vi "EOL TCP Connection Manager.vi"(8 "error in":errorcluster, 10 "VI Ref":refnum<vi>, 11 "thread queue":refnum<queue>) -> (0 "error out":errorcluster)   [LabVIEW 2012, in "tcp connection.lvclass"]
doc: "acts as a server for a single networked hmi"
uses:
  classes/connection/tcp connection.lvclass
  classes/server side connection/tcp server connection.lvclass
  typedefs/tcp connection info.ctl
  typedefs/connection type.ctl
  interthread comms/typedefs/app type.ctl
  typedefs/interapp tx message request.ctl
  interthread comms/typedefs/interthread message.ctl
  typedefs/interapp message.ctl
  typedefs/interthread get connection status message.ctl
  typedefs/interthread connection status response.ctl
  interthread comms/typedefs/HMI PC thread IDs.ctl
  typedefs/interapp message actions.ctl
  interthread comms/typedefs/state queue fglbl actions.ctl
  interthread comms/typedefs/station cDAQ thread IDs.ctl
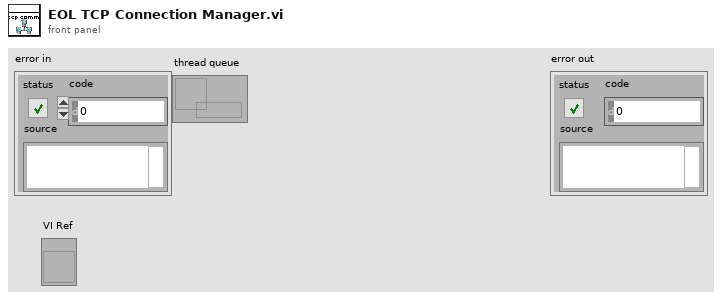
[diagram p1: front panel]
types:
  T1 = typedef "tcp connection info.ctl" = cluster{"server ip address":string, "server port":i32, "connection type":T2}
  T2 = typedef "connection type.ctl" = enum16{"client", "server"}
  T3 = cluster{"connections":refnum<class "tcp connection.lvclass">[]}
  T4 = typedef "station cDAQ thread IDs.ctl" = enum16{"cDAQ main", "analog input", "eol test exe", "nvh test exe", "tcp comms"}
  T5 = typedef "interapp message actions.ctl" = enum16{"init", "request message tx"}
  T6 = typedef "interthread message.ctl" = cluster{"destination state":string, "data":variant}
  T7 = typedef "HMI PC thread IDs.ctl" = enum16{"hmi main", "file output", "tcp comms", "NVH process"}
  T8 = typedef "state queue fglbl actions.ctl" = enum16{"init queues", "get queue ref", "destroy queues"}
  T9 = typedef "interthread get connection status message.ctl" = cluster{"tcp connection info":T1, "reply-to state":string, "reply-to thread":string, "reply-to app":T10}
  T10 = typedef "app type.ctl" = enum16{"PC", "cDAQ", "AuditHMI"}
  T11 = typedef "interthread connection status response.ctl" = cluster{"tcp connection info":T1, "connected":bool}
  T12 = typedef "interapp tx message request.ctl" = cluster{"destination app":T10, "destination thread":string, "tcp connection info":T1, "message":T6}
  T13 = typedef "interapp message.ctl" = cluster{"destination app":T10, "destination thread":string, "message":T6}
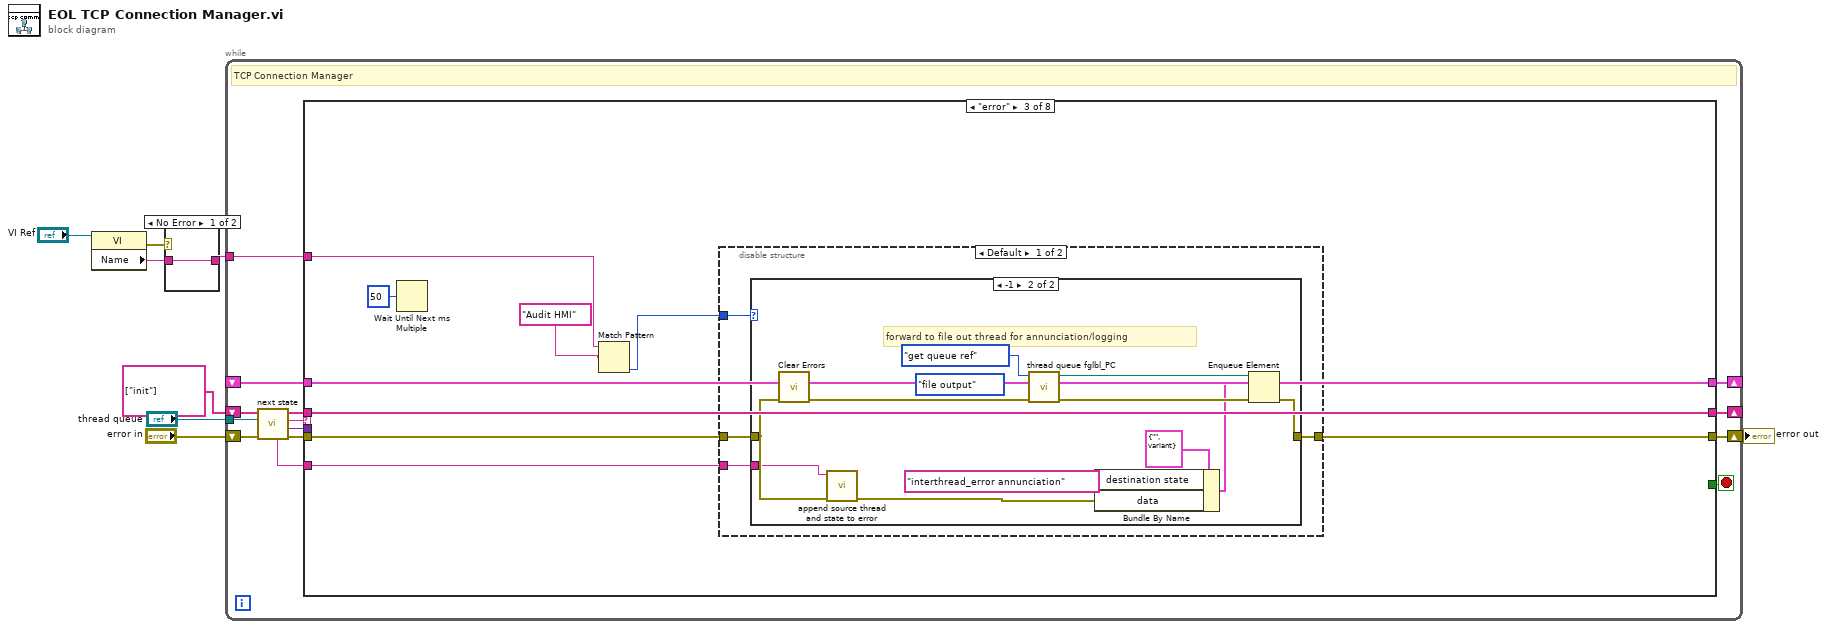
[diagram p0: block diagram]
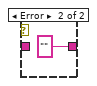
[diagram p2: hidden frame]
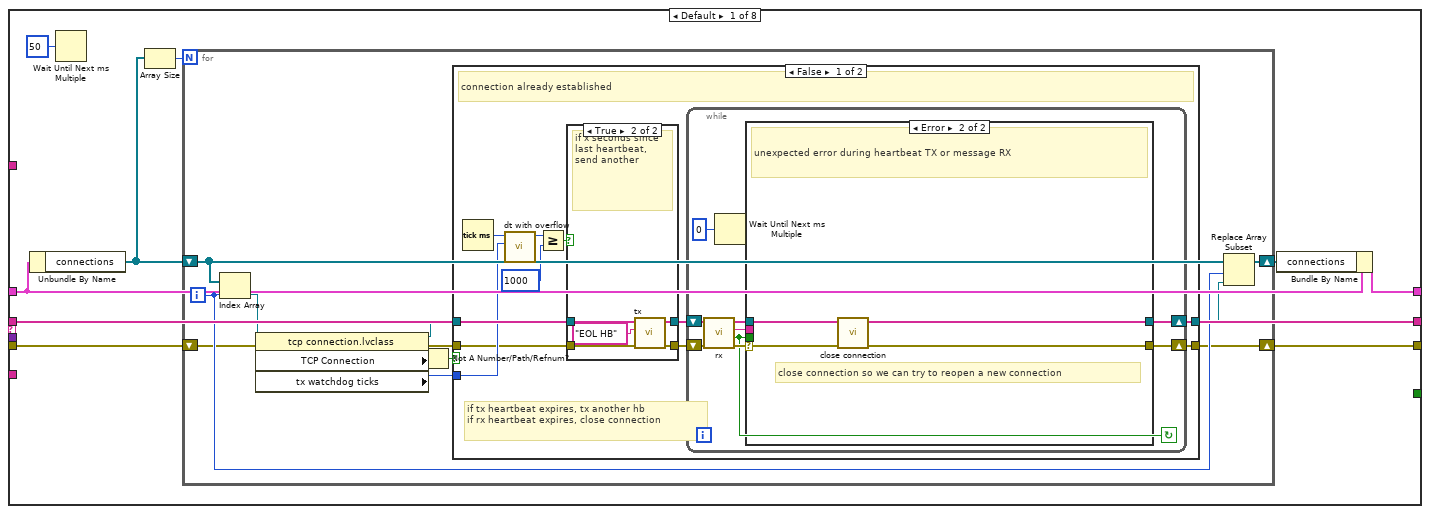
[diagram p3: hidden frame]
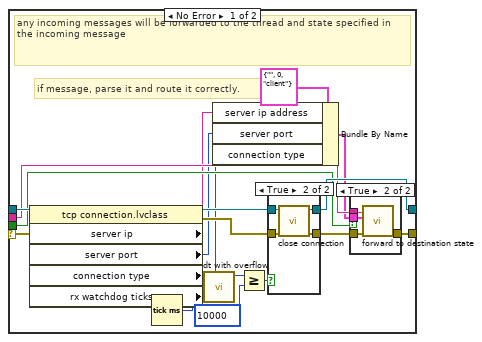
[diagram p4: hidden frame]
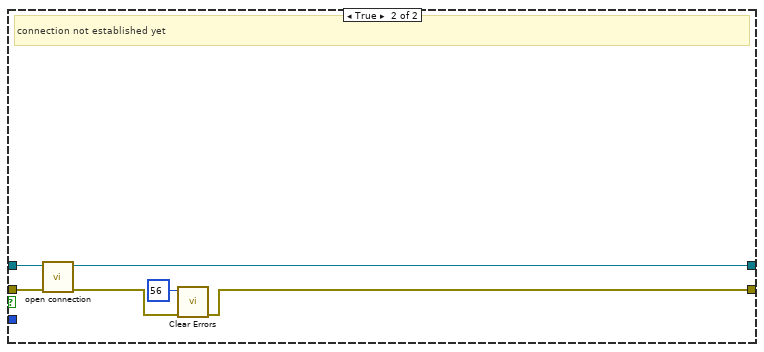
[diagram p8: hidden frame]
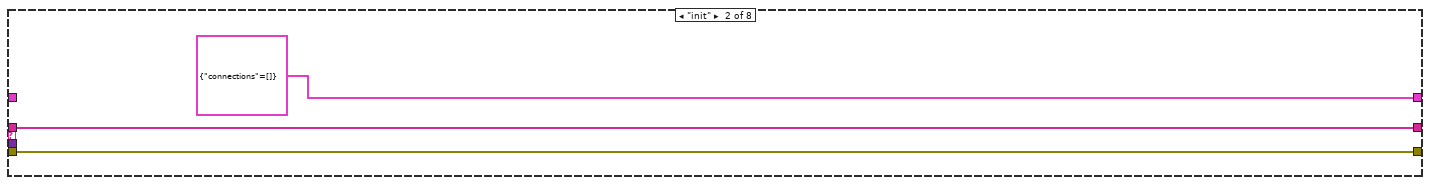
[diagram p9: hidden frame]
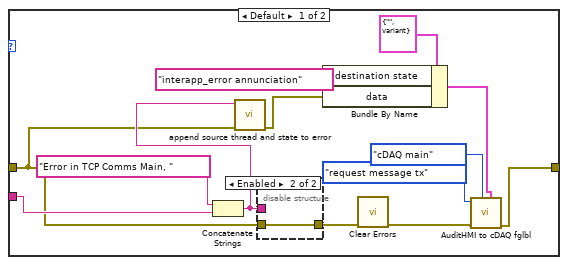
[diagram p10: hidden frame]
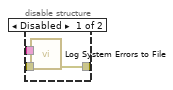
[diagram p11: hidden frame]
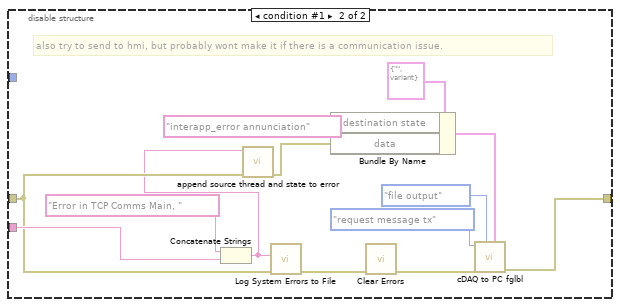
[diagram p12: hidden frame]
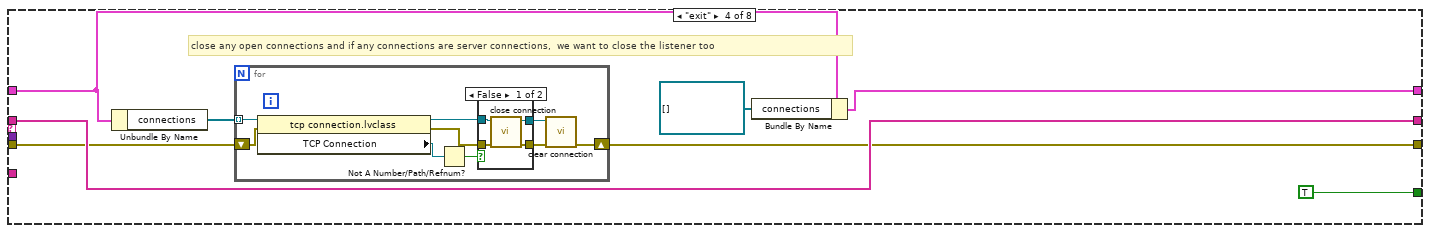
[diagram p13: hidden frame]
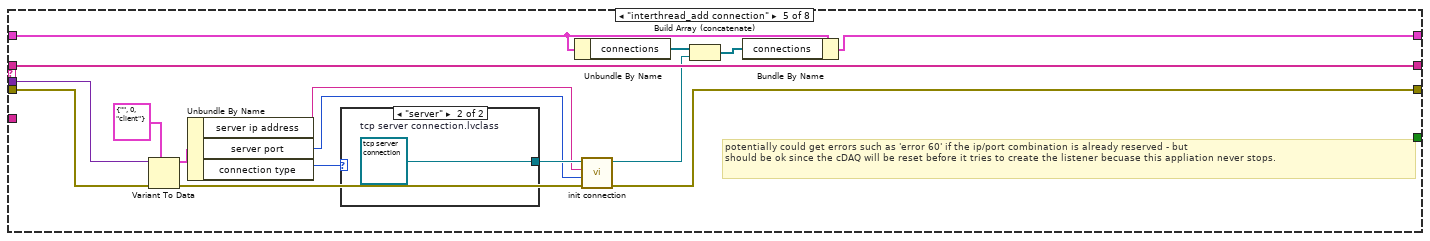
[diagram p15: hidden frame]
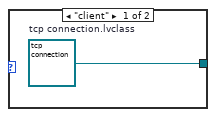
[diagram p16: hidden frame]
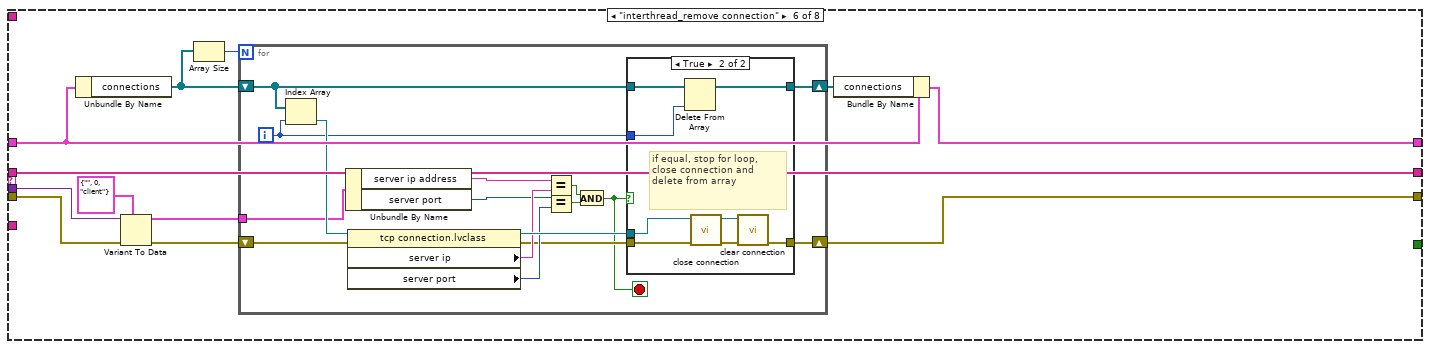
[diagram p17: hidden frame]
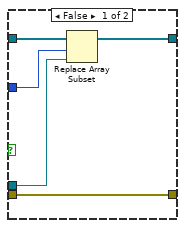
[diagram p18: hidden frame]
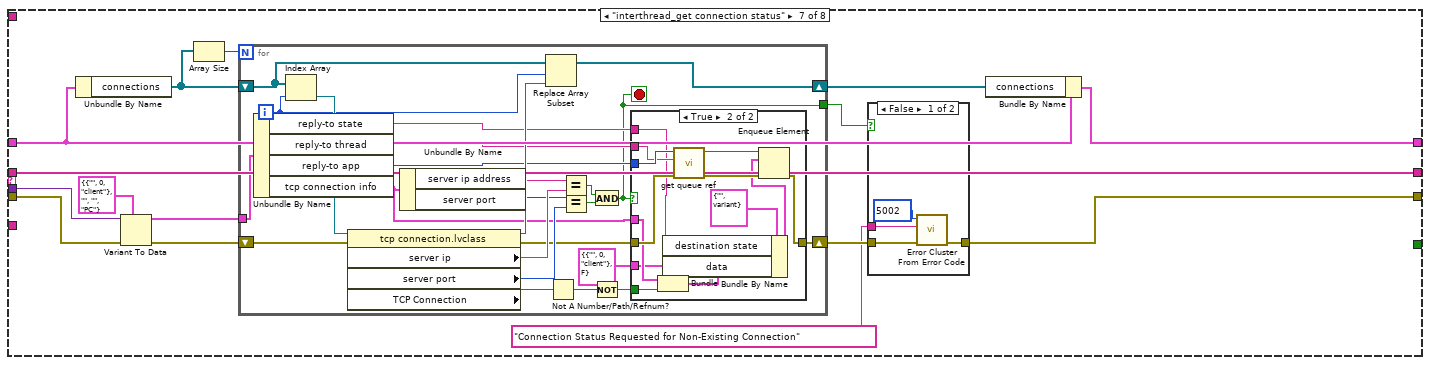
[diagram p19: hidden frame]
diagram:
  n1 = property class="VI"(reference="VI Ref") -> (error out=w3:errorcluster, "Name"=w1:string)  [unwired: 1 in, 1 out]
  n2 = case shown="No Error" w3 {
    tunnel: [w9 "" ("Name")] -> w2
    tunnel: w1 -> [w9 _]
    frame No Error {
    }
    frame Error {
    }
  }
  n3 = while {
    shift-right: [w23] -> _
    shift-left: _ -> [w24]
    shift-right: [w19] -> _
    shift-left: string[] ["init"] ("event queue out") -> [w22]
    shift-right: [w14] -> w7
    shift-left: "error in" -> [w18]
    tunnel: "thread queue" -> [w15]
    tunnel: w2 -> [w11]
    stop <- w16 stop-if-true
    # "TCP Connection Manager"
    n4 = call "next state.vi"("error in"=w18, "thread queue"=w15, "state queue in"=w22) -> ("error out"=w17:errorcluster, "data"=w13:variant, "next state"=w21:string, "state queue out"=w20:string[], "previous state"=w12:string)  [unwired: 4 in]
    n5 = case shown="\"error\"" w21 {
      tunnel: w24 -> [w26 _ w123 w171 w204 w215 w260 w316]
      tunnel: [w28 T3 {"connections"=[]} w123 w177 w203 w214 w259 w315] -> w23
      tunnel: w20 -> [w33 w115 w122 w178 w209 w223 w267 w323]
      tunnel: [w33 w115 w122 w178 w209 w223 w267 w323] -> w19
      tunnel: w17 -> [w29 w113 w116 w174 w208 w221 w265 w321]
      tunnel: [w25 w113 w121 w173 w198 w213 w255 w314] -> w14
      tunnel: [_ _ _ TRUE _ _ _ _] -> w16
      tunnel: w13 -> [_ _ _ _ w207 w222 w266 w322]
      tunnel: w12 -> [_ _ w120 _ _ _ _ _]
      tunnel: w11 -> [_ _ w118 _ _ _ _ _]
      frame Default {
        n6 = Unbundle By Name(w26) -> ("connections"=w30:refnum<class "tcp connection.lvclass">[])
        n7 = Wait Until Next ms Multiple(millisecond multiple=u32 50) -> ()  [unwired: 1 out]
        n8 = Array Size(array=w30) -> (size(s)=w31:i32)
        n9 = for {
          N: w31 -> [_]
          shift-right: [w40] -> w25
          shift-left: w29 -> [w38]
          shift-right: [w44] -> w27
          shift-left: w30 -> [w41]
          i -> [w42]
          n10 = Index Array(array=w41, index=w42) -> (element=w39:refnum<class "tcp connection.lvclass">)
          n11 = property class="tcp connection.lvclass"(reference=w39, error in=w38) -> (reference out=w36:refnum<class "tcp connection.lvclass">, error out=w37:errorcluster, "TCP Connection"=w35:refnum<k5>, "tx watchdog ticks"=w34:u32)
          n12 = Not A Number/Path/Refnum?(number/path/refnum=w35) -> (NaN/Path/Refnum?=w45:bool)
          n13 = case shown="False" w45 {
            tunnel: w37 -> [w52 w111]
            tunnel: [w47 w107] -> w40
            tunnel: w36 -> [w53 w112]
            tunnel: [w46 w110] -> w43
            tunnel: w34 -> [w54 _]
            frame False {
              # "if tx heartbeat expires, tx another hb\nif rx heartbeat expires, close connection"
              # "connection already established"
              n14 = Tick Count (ms)() -> (millisecond timer value=w50:u32)
              n15 = call "dt with overflow.vi"("t0"=w54, "t1"=w50) -> ("t1-t0"=w56:u32)  [unwired: 9 in]
              n16 = Greater Or Equal?(x=w56, y=u32 1000) -> (x >= y?=w55:bool)
              n17 = case shown="True" w55 {
                tunnel: w52 -> [w101 w106]
                tunnel: [w101 w103] -> w49
                tunnel: w53 -> [w100 w105]
                tunnel: [w100 w104] -> w48
                frame False {
                }
                frame True {
                  # "if x seconds since last heartbeat, send another"
                  n18 = call-dynamic "tx.vi"("error in (no error)"=w106, "tx"="EOL HB", "tcp server in"=w105) -> ("error out"=w103:errorcluster, "tcp server out"=w104:refnum<class "tcp connection.lvclass">)  [unwired: 7 in]
                }
              }
              n19 = while {
                shift-right: [w59] -> w47
                shift-left: w49 -> [w65]
                shift-right: [w62] -> w46
                shift-left: w48 -> [w64]
                stop <- w58 continue-if-true
                n20 = call-dynamic "rx.vi"("error in (no error)"=w65, "tcp server in"=w64) -> ("error out"=w61:errorcluster, "new message"=w58:bool, "rx"=w60:string, "tcp server out"=w63:refnum<class "tcp connection.lvclass">)  [unwired: 6 in]
                n21 = Wait Until Next ms Multiple(millisecond multiple=u32 0) -> ()  [unwired: 1 out]
                n22 = case shown="Error" w61 {
                  selector: w61 -> [w77 w98]
                  tunnel: w63 -> [w82 w99]
                  tunnel: [w73 w96] -> w59
                  tunnel: [w78 w97] -> w62
                  tunnel: w60 -> [w75 _]
                  tunnel: w58 -> [w76 _]
                  frame No Error {
                    # "if message, parse it and route it correctly."
                    # "any incoming messages will be forwarded to the thread and state specified in the incoming message"
                    n23 = property class="tcp connection.lvclass"(reference=w82, error in=w77) -> (reference out=w79:refnum<class "tcp connection.lvclass">, error out=w80:errorcluster, "server ip"=w68:string, "server port"=w67:i32, "connection type"=w66:T2, "rx watchdog ticks"=w72:u32)
                    n24 = Tick Count (ms)() -> (millisecond timer value=w69:u32)
                    n25 = call "dt with overflow.vi"("t0"=w72, "t1"=w69) -> ("t1-t0"=w84:u32)  [unwired: 9 in]
                    n26 = Bundle By Name(cluster=T1 {"server ip address"="", "server port"=0, "connection type"=enum."client"} ("message source"), "server ip address"=w68, "server port"=w67, "connection type"=w66) -> (w70:T1)
                    n27 = Greater Or Equal?(x=w84, y=u32 10000) -> (x >= y?=w81:bool)
                    n28 = case shown="True" w81 {
                      tunnel: w80 -> [w91 w95]
                      tunnel: [w91 w94] -> w74
                      tunnel: w79 -> [w90 w93]
                      tunnel: [w90 w92] -> w78
                      frame False {
                      }
                      frame True {
                        n29 = call "close connection.vi"("error in (no error)"=w95, "tcp server in"=w93) -> ("error out"=w94:errorcluster, "tcp server out"=w92:refnum<class "tcp connection.lvclass">)  [unwired: 8 in]
                      }
                    }
                    n30 = case shown="True" w76 {
                      tunnel: w75 -> [_ w87]
                      tunnel: w74 -> [w85 w88]
                      tunnel: [w85 w89] -> w73
                      tunnel: w70 -> [_ w86]
                      frame False {
                      }
                      frame True {
                        n31 = call "forward to destination state.vi"("error in (no error)"=w88, "message source"=w86, "rx"=w87) -> ("error out"=w89:errorcluster)  [unwired: 8 in]
                      }
                    }
                  }
                  frame Error {
                    # "close connection so we can try to reopen a new connection"
                    # "unexpected error during heartbeat TX or message RX"
                    n32 = call "close connection.vi"("error in (no error)"=w98, "tcp server in"=w99) -> ("error out"=w96:errorcluster, "tcp server out"=w97:refnum<class "tcp connection.lvclass">)  [unwired: 8 in]
                  }
                }
              }
            }
            frame True {
              # "connection not established yet"
              n33 = call-dynamic "open connection.vi"("error in (no error)"=w111, "tcp connection in"=w112) -> ("error out"=w108:errorcluster, "tcp connection out"=w110:refnum<class "tcp connection.lvclass">)  [unwired: 8 in]
              n34 = call <vilib>:"Clear Errors.vi"("error in (no error)"=w108, "specific error code to clear (0: all)"=56) -> ("error out"=w107:errorcluster)  [unwired: 4 in, 1 out]
            }
          }
          n35 = Replace Array Subset(array=w41, new element=w43, index=w42) -> (w44:refnum<class "tcp connection.lvclass">[])
        }
        n36 = Bundle By Name(cluster=w26, "connections"=w27) -> (w28:T3)
      }
      frame "init" {
      }
      frame "error" {
        n37 = Wait Until Next ms Multiple(millisecond multiple=u32 50) -> ()  [unwired: 1 out]
        n38 = Match Pattern(string=w118, regular expression="Audit HMI") -> (offset past match=w119:i32)  [unwired: 1 in, 3 out]
        n39 = disable-structure shown="Default" {
          disable-tunnel: [w128 w162] -> w121
          disable-tunnel: w116 -> [w127 w160]
          disable-tunnel: w120 -> [w126 w161]
          disable-tunnel: w119 -> [w125 _]
          frame condition #0 (active) {
            n40 = case shown="-1" w125 {
              tunnel: [w129 w150] -> w128
              tunnel: w127 -> [w134 w148]
              tunnel: w126 -> [w135 w146]
              frame Default {
                n41 = Concatenate Strings("Error in TCP Comms Main, " ("Comments"), w135) -> (w136:string)
                n42 = call "append source thread and state to error.vi"("error in (no error)"=w134, "String"=w136) -> ("error out"=w137:errorcluster)  [unwired: 9 in]
                n43 = disable-structure shown="Enabled" {
                  disable-tunnel: [w144 w145] -> w138
                  disable-tunnel: w136 -> [w143 _]
                  disable-tunnel: w134 -> [w142 w145]
                  frame Disabled {
                    n44 = call "Log System Errors to File.vi"("error in"=w142, "Comments"=w143) -> ("error out"=w144:errorcluster)  [unwired: 1 in, 8 out]
                  }
                  frame Enabled {
                  }
                }
                n45 = Bundle By Name(cluster=T6 {"destination state"="", "data"=variant} ("message"), "destination state"="interapp_error annunciation", "data"=w137) -> (w132:T6)
                n46 = call <vilib>:"Clear Errors.vi"("error in (no error)"=w138) -> ("error out"=w133:errorcluster)  [unwired: 5 in, 1 out]
                n47 = call "AuditHMI to cDAQ fglbl.vi"("message"=w132, "Station cDAQ Thread ID"=station_cDAQ_thread_IDs."cDAQ main", "error in (no error)"=w133, "action"=interapp_message_actions."request message tx") -> ("error out"=w129:errorcluster)  [unwired: 7 in]
              }
              frame -1 {
                # "forward to file out thread for annunciation/logging"
                n48 = call <vilib>:"Clear Errors.vi"("error in (no error)"=w148) -> ("error out"=w157:errorcluster)  [unwired: 5 in, 1 out]
                n49 = call "append source thread and state to error.vi"("error in (no error)"=w148, "String"=w146) -> ("error out"=w147:errorcluster)  [unwired: 9 in]
                n50 = call "thread queue fglbl_PC.vi"("error in (no error)"=w157, "Station cDAQ Thread Queue"=HMI_PC_thread_IDs."file output", "action"=state_queue_fglbl_actions."get queue ref") -> ("error out"=w154:errorcluster, "queue out"=w153:refnum<queue>)  [unwired: 6 in, 1 out]
                n51 = Bundle By Name(cluster=T6 {"destination state"="", "data"=variant} ("message"), "destination state"="interthread_error annunciation", "data"=w147) -> (w149:T6)
                n52 = Enqueue Element(queue=w153, element=w149, error in (no error)=w154) -> (error out=w150:errorcluster)  [unwired: 1 in, 2 out]
              }
            }
          }
          frame condition #1 {
            # "also try to send to hmi, but probably wont make it if there is a communication issue."
            n53 = Concatenate Strings("Error in TCP Comms Main, " ("Comments"), w161) -> (w158:string)
            n54 = call "append source thread and state to error.vi"("error in (no error)"=w160, "String"=w158) -> ("error out"=w159:errorcluster)  [unwired: 9 in]
            n55 = call "Log System Errors to File.vi"("error in"=w160, "Comments"=w158) -> ("error out"=w164:errorcluster)  [unwired: 1 in, 8 out]
            n56 = Bundle By Name(cluster=T6 {"destination state"="", "data"=variant} ("message"), "destination state"="interapp_error annunciation", "data"=w159) -> (w170:T6)
            n57 = call <vilib>:"Clear Errors.vi"("error in (no error)"=w164) -> ("error out"=w163:errorcluster)  [unwired: 5 in, 1 out]
            n58 = call "cDAQ to PC fglbl.vi"("message"=w170, "PC HMI Thread"=HMI_PC_thread_IDs."file output" ("PC HMI Thread Queues"), "error in (no error)"=w163, "action"=interapp_message_actions."request message tx") -> ("error out"=w162:errorcluster)  [unwired: 7 in]
          }
        }
      }
      frame "exit" {
        # "close any open connections and if any connections are server connections,  we want to close the listener too"
        n59 = Unbundle By Name(w171) -> ("connections"=w175:refnum<class "tcp connection.lvclass">[])
        n60 = for {
          tunnel: w175 -> [w184] mode=indexing
          shift-right: [w186] -> w173
          shift-left: w174 -> [w183]
          n61 = property class="tcp connection.lvclass"(reference=w184, error in=w183) -> (reference out=w182:refnum<class "tcp connection.lvclass">, error out=w181:errorcluster, "TCP Connection"=w180:refnum<k5>)
          n62 = Not A Number/Path/Refnum?(number/path/refnum=w180) -> (NaN/Path/Refnum?=w179:bool)
          n63 = case shown="False" w179 {
            tunnel: [w191 w192] -> w187
            tunnel: [w190 w193] -> w185
            tunnel: w182 -> [w189 w193]
            tunnel: w181 -> [w188 w192]
            frame False {
              n64 = call "close connection.vi"("error in (no error)"=w188, "tcp server in"=w189) -> ("error out"=w191:errorcluster, "tcp server out"=w190:refnum<class "tcp connection.lvclass">)  [unwired: 8 in]
            }
            frame True {
            }
          }
          n65 = call-dynamic "clear connection.vi"("error in (no error)"=w187, "tcp server in"=w185) -> ("error out"=w186:errorcluster)  [unwired: 8 in, 1 out]
        }
        n66 = Bundle By Name(cluster=w171, "connections"=refnum<class "tcp connection.lvclass">[] []) -> (w177:T3)
      }
      frame "interthread_add connection" {
        # "potentially could get errors such as 'error 60' if the ip/port combination is already reserved - but\nshould be ok since the cDAQ will be reset before it tries to create the listener becuase this appliation never stops."
        n67 = Variant To Data(error in=w208, type=T1 {"server ip address"="", "server port"=0, "connection type"=enum."client"} ("tcp connection info"), Variant=w207) -> (data=w201:T1, error out=w199:errorcluster)
        n68 = Unbundle By Name(w201) -> ("server ip address"=w196:string, "server port"=w195:i32, "connection type"=w200:T2)
        n69 = case shown="\"server\"" w200 {
          tunnel: [w210 w211] -> w197
          frame "client" {
            w210 = refnum<class "tcp connection.lvclass"> refnum  # tcp connection.lvclass
          }
          frame "server" {
            w211 = refnum<class "tcp server connection.lvclass"> refnum  # tcp server connection.lvclass
          }
        }
        n70 = Unbundle By Name(w204) -> ("connections"=w206:refnum<class "tcp connection.lvclass">[])
        n71 = call-dynamic "init connection.vi"("error in (no error)"=w199, "server port"=w195, "server ip"=w196, "tcp connection in"=w197) -> ("error out"=w198:errorcluster, "tcp connection out"=w194:refnum<class "tcp connection.lvclass">)  [unwired: 6 in]
        n72 = Build Array (concatenate)(w206, w194) -> (w205:refnum<class "tcp connection.lvclass">[])
        n73 = Bundle By Name(cluster=w204, "connections"=w205) -> (w203:T3)
      }
      frame "interthread_remove connection" {
        n74 = Unbundle By Name(w215) -> ("connections"=w218:refnum<class "tcp connection.lvclass">[])
        n75 = Variant To Data(error in=w221, type=T1 {"server ip address"="", "server port"=0, "connection type"=enum."client"} ("tcp connection info"), Variant=w222) -> (data=w212:T1, error out=w217:errorcluster)
        n76 = Array Size(array=w218) -> (size(s)=w219:i32)
        n77 = for {
          N: w219 -> [_]
          shift-right: [w235] -> w216
          shift-left: w218 -> [w238]
          shift-right: [w226] -> w213
          shift-left: w217 -> [w234]
          tunnel: w212 -> [w233]
          i -> [w237]
          stop <- w224 stop-if-true
          n78 = Index Array(array=w238, index=w237) -> (element=w239:refnum<class "tcp connection.lvclass">)
          n79 = Unbundle By Name(w233) -> ("server ip address"=w232:string, "server port"=w230:i32)
          n80 = property class="tcp connection.lvclass"(reference=w239, error in=w234) -> (reference out=w236:refnum<class "tcp connection.lvclass">, error out=w225:errorcluster, "server ip"=w231:string, "server port"=w229:i32)
          n81 = Equal?(x=w232, y=w231) -> (x = y?=w228:bool)
          n82 = Equal?(x=w230, y=w229) -> (x = y?=w227:bool)
          n83 = And(x=w228, y=w227) -> (x .and. y?=w224:bool)
          n84 = case shown="True" w224 {
            tunnel: w238 -> [w244 w250]
            tunnel: w237 -> [w243 w248]
            tunnel: w236 -> [w242 w251]
            tunnel: [w241 w249] -> w235
            tunnel: [w240 w245] -> w226
            tunnel: w225 -> [w240 w252]
            frame False {
              n85 = Replace Array Subset(array=w244, new element=w242, index=w243) -> (w241:refnum<class "tcp connection.lvclass">[])
            }
            frame True {
              # "if equal, stop for loop,\nclose connection and\ndelete from array"
              n86 = Delete From Array(array=w250, index=w248) -> (array with subset deleted=w249:refnum<class "tcp connection.lvclass">[])  [unwired: 1 in, 1 out]
              n87 = call "close connection.vi"("error in (no error)"=w252, "tcp server in"=w251) -> ("error out"=w246:errorcluster, "tcp server out"=w247:refnum<class "tcp connection.lvclass">)  [unwired: 8 in]
              n88 = call-dynamic "clear connection.vi"("error in (no error)"=w246, "tcp server in"=w247) -> ("error out"=w245:errorcluster)  [unwired: 8 in, 1 out]
            }
          }
        }
        n89 = Bundle By Name(cluster=w215, "connections"=w216) -> (w214:T3)
      }
      frame "interthread_get connection status" {
        n90 = Unbundle By Name(w260) -> ("connections"=w263:refnum<class "tcp connection.lvclass">[])
        n91 = Variant To Data(error in=w265, type=T9 {"tcp connection info"={"server ip address"="", "server port"=0, "connection type"=enum."client"}, "reply-to state"="", "reply-to thread"="", "reply-to app"=enum."PC"}, Variant=w266) -> (data=w258:T9, error out=w262:errorcluster)
        n92 = Array Size(array=w263) -> (size(s)=w264:i32)
        n93 = for {
          N: w264 -> [_]
          shift-right: [w292] -> w261
          shift-left: w263 -> [w295]
          shift-right: [w281] -> w254
          shift-left: w262 -> [w291]
          tunnel: w258 -> [w290]
          tunnel: [w278] -> w256
          i -> [w294]
          stop <- w278 stop-if-true
          n94 = Unbundle By Name(w290) -> ("reply-to state"=w279:string, "reply-to thread"=w280:string, "reply-to app"=w283:T10, "tcp connection info"=w275:T1)
          n95 = Index Array(array=w295, index=w294) -> (element=w296:refnum<class "tcp connection.lvclass">)
          n96 = property class="tcp connection.lvclass"(reference=w296, error in=w291) -> (reference out=w293:refnum<class "tcp connection.lvclass">, error out=w282:errorcluster, "server ip"=w289:string, "server port"=w288:i32, "TCP Connection"=w285:refnum<k5>)
          n97 = Unbundle By Name(w275) -> ("server ip address"=w277:string, "server port"=w276:i32)
          n98 = Replace Array Subset(array=w295, new element=w293, index=w294) -> (w292:refnum<class "tcp connection.lvclass">[])
          n99 = Not A Number/Path/Refnum?(number/path/refnum=w285) -> (NaN/Path/Refnum?=w284:bool)
          n100 = Equal?(x=w277, y=w289) -> (x = y?=w287:bool)
          n101 = Equal?(x=w276, y=w288) -> (x = y?=w286:bool)
          n102 = And(x=w287, y=w286) -> (x .and. y?=w278:bool)
          n103 = Not(x=w284) -> (.not. x?=w273:bool)
          n104 = case shown="True" w278 {
            tunnel: w273 -> [_ w301]
            tunnel: w283 -> [_ w310]
            tunnel: w282 -> [w297 w309]
            tunnel: [w297 w306] -> w281
            tunnel: w280 -> [_ w304]
            tunnel: w279 -> [_ w303]
            tunnel: w275 -> [_ w300]
            tunnel: T11 {"tcp connection info"={"server ip address"="", "server port"=0, "connection type"=enum."client"}, "connected"=FALSE} ("cluster") -> [_ w298]
            frame False {
            }
            frame True {
              n105 = Bundle(cluster=w298, "tcp connection info"=w300, "connected"=w301) -> (w299:T11)
              n106 = Bundle By Name(cluster=T6 {"destination state"="", "data"=variant} ("message"), "destination state"=w303, "data"=w299) -> (w302:T6)
              n107 = call "get queue ref.vi"("error in (no error)"=w309, "destination thread"=w304, "destination app type"=w310) -> ("error out"=w307:errorcluster, "queue ref"=w308:refnum<queue>)  [unwired: 7 in]
              n108 = Enqueue Element(queue=w308, element=w302, error in (no error)=w307) -> (error out=w306:errorcluster)  [unwired: 1 in, 2 out]
            }
          }
        }
        n109 = case shown="False" w256 {
          tunnel: [w271 w272] -> w255
          tunnel: w254 -> [w270 w272]
          tunnel: "Connection Status Requested for Non-Existing Connection" -> [w269 _]
          frame False {
            n110 = call <vilib>:"Error Cluster From Error Code.vi"("error in (no error)"=w270, "error message (\"\")"=w269, "error code (0)"=5002) -> ("error out"=w271:errorcluster)  [unwired: 6 in]
          }
          frame True {
          }
        }
        n111 = Bundle By Name(cluster=w260, "connections"=w261) -> (w259:T3)
      }
      frame "interthread_tx" {
        n112 = Unbundle By Name(w316) -> ("connections"=w319:refnum<class "tcp connection.lvclass">[])
        n113 = Wait Until Next ms Multiple(millisecond multiple=u32 0) -> ()  [unwired: 1 out]
        n114 = Variant To Data(error in=w321, type=T12 {"destination app"=enum."PC", "destination thread"="", "tcp connection info"={"server ip address"="", "server port"=0, "connection type"=enum."client"}, "message"={"destination state"="", "data"=variant}}, Variant=w322) -> (data=w313:T12, error out=w318:errorcluster)
        n115 = Array Size(array=w319) -> (size(s)=w320:i32)
        n116 = for {
          N: w320 -> [_]
          shift-right: [w342] -> w317
          shift-left: w319 -> [w344]
          shift-right: [w330] -> w314
          shift-left: w318 -> [w341]
          tunnel: w313 -> [w340]
          i -> [w343]
          stop <- w333 stop-if-true
          n117 = Index Array(array=w344, index=w343) -> (element=w345:refnum<class "tcp connection.lvclass">)
          n118 = Unbundle By Name(w340) -> ("destination app"=w328:T10, "destination thread"=w327:string, "message"=w326:T6, "tcp connection info.server ip address"=w339:string, "tcp connection info.server port"=w337:i32)
          n119 = property class="tcp connection.lvclass"(reference=w345, error in=w341) -> (reference out=w331:refnum<class "tcp connection.lvclass">, error out=w329:errorcluster, "server ip"=w338:string, "server port"=w336:i32, "TCP Connection"=w325:refnum<k5>)
          n120 = Not A Number/Path/Refnum?(number/path/refnum=w325) -> (NaN/Path/Refnum?=w324:bool)
          n121 = Equal?(x=w339, y=w338) -> (x = y?=w335:bool)
          n122 = Equal?(x=w337, y=w336) -> (x = y?=w334:bool)
          n123 = Compound Arithmetic op=AND(w335, w334, invert w324) -> (w333:bool)
          n124 = case shown="True" w333 {
            tunnel: [w347 w356] -> w332
            tunnel: w331 -> [w347 w358]
            tunnel: [w346 w359] -> w330
            tunnel: w329 -> [w346 w351]
            tunnel: w328 -> [_ w354]
            tunnel: w327 -> [_ w353]
            tunnel: w326 -> [_ w352]
            frame False {
            }
            frame True {
              # "found connection and it has been established, tx"
              n125 = Bundle By Name(cluster=T13 {"destination app"=enum."PC", "destination thread"="", "message"={"destination state"="", "data"=variant}} ("interapp tx request"), "destination app"=w354, "destination thread"=w353, "message"=w352) -> (w348:T13)
              n126 = Flatten To String(anything=w348, error in (no error)=w351) -> (data string=w349:string, error out=w350:errorcluster)  [unwired: 2 in, 1 out]
              n127 = call-dynamic "tx.vi"("error in (no error)"=w350, "tx"=w349, "tcp server in"=w358) -> ("error out"=w360:errorcluster, "tcp server out"=w357:refnum<class "tcp connection.lvclass">)  [unwired: 7 in]
              n128 = case shown="Error" w360 {
                selector: w360 -> [w361 w366]
                tunnel: [w361 w365] -> w359
                tunnel: w357 -> [w362 w364]
                tunnel: [w362 w363] -> w356
                frame No Error {
                }
                frame Error {
                  n129 = call "close connection.vi"("error in (no error)"=w366, "tcp server in"=w364) -> ("error out"=w365:errorcluster, "tcp server out"=w363:refnum<class "tcp connection.lvclass">)  [unwired: 8 in]
                }
              }
            }
          }
          n130 = Replace Array Subset(array=w344, new element=w332, index=w343) -> (w342:refnum<class "tcp connection.lvclass">[])
        }
        n131 = Bundle By Name(cluster=w316, "connections"=w317) -> (w315:T3)
      }
    }
  }
  "error out" <- w7
